vi "Ridders Zero Inner Part.vi"(0 "start/end/f(x)":T1 {"end" format="%.2f"; "start" format="%.2f"; "y value copy" format="%.2f"; "y value" format="%.2f"}, 1 "list of variables":i32[](array[numeric]), 2 "table":i32[][](array[numeric]), 3 "result":dbl[](array[numeric]) format="%.2f", 4 "accuracy":dbl format="%.2f", 5 "case":bool) -> (6 "y value":dbl format="%.2f", 7 "end":dbl format="%.2f", 8 "error":i32)   [LabVIEW 2010, in "NI_Gmath.lvlib"]
uses:
  NI_Gmath.lvlib
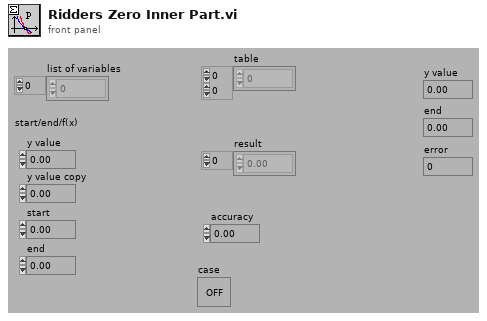
[diagram p1: front panel]
types:
  T1 = cluster{"y value":dbl, "y value copy":dbl, "start":dbl, "end":dbl}
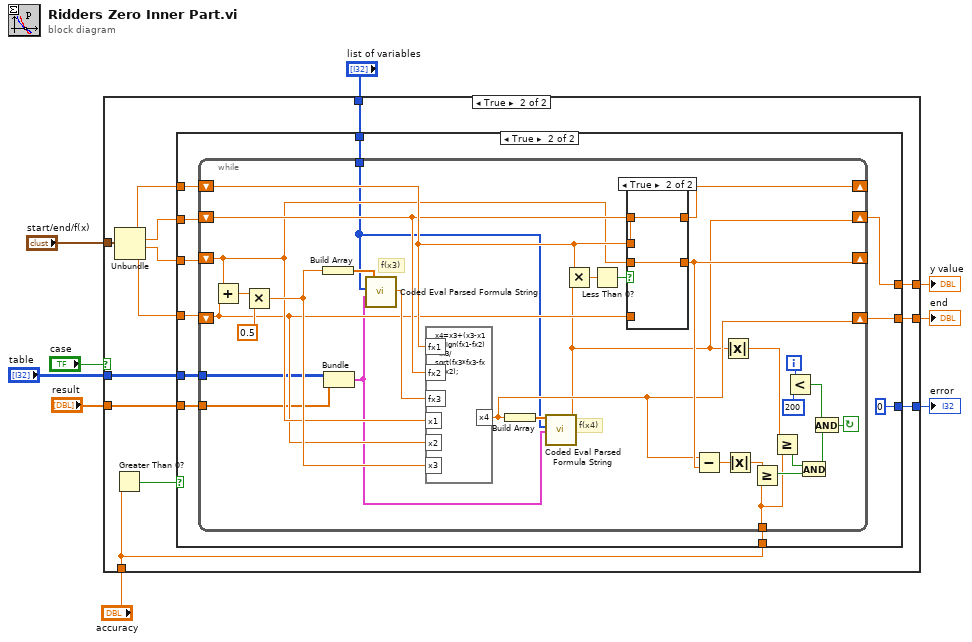
[diagram p0: block diagram]
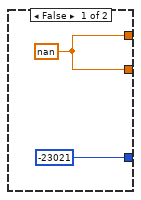
[diagram p2: hidden frame]
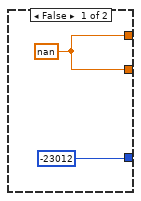
[diagram p3: hidden frame]
diagram:
  n1 = case shown="True" "case" {
    tunnel: [-23021 w23] -> w2
    tunnel: "accuracy" -> [_ w17]
    tunnel: [w10 w22] -> w4
    tunnel: [w10 w21] -> w5
    tunnel: "list of variables" -> [_ w20]
    tunnel: "table" -> [_ w19]
    tunnel: "result" -> [_ w18]
    tunnel: "start/end/f(x)" -> [_ w16]
    frame False {
      w10 = nan
    }
    frame True {
      n2 = Greater Than 0?(x=w17) -> (x > 0?=w24:bool)
      n3 = Unbundle(w16) -> ("y value"=w12:dbl, "y value copy"=w13:dbl, "start"=w14:dbl, "end"=w15:dbl)
      n4 = case shown="True" w24 {
        tunnel: w17 -> [_ w37]
        tunnel: w12 -> [_ w36]
        tunnel: w13 -> [_ w35]
        tunnel: w14 -> [_ w34]
        tunnel: w15 -> [_ w33]
        tunnel: [-23012 0] -> w23
        tunnel: [w25 w31] -> w22
        tunnel: [w25 w30] -> w21
        tunnel: w20 -> [_ w29]
        tunnel: w19 -> [_ w28]
        tunnel: w18 -> [_ w27]
        frame False {
          w25 = nan
        }
        frame True {
          n5 = while {
            tunnel: w27 -> [w39]
            tunnel: w28 -> [w41]
            tunnel: w29 -> [w40]
            tunnel: w37 -> [w51]
            shift-left: w35 -> [w62]
            shift-right: [w38] -> w30
            shift-left: w36 -> [w64]
            shift-right: [w63] -> _
            shift-left: w33 -> [w52]
            shift-right: [w50] -> w31
            shift-left: w34 -> [w53]
            shift-right: [w61] -> _
            i -> [w49]
            stop <- w46 continue-if-true
            # "f(x4)"
            # "f(x3)"
            n6 = Add(x=w53, y=w52) -> (x+y=w67:dbl)
            n7 = Multiply(x=w67, y=0.5) -> (x*y=w54:dbl)
            n8 = Build Array(w54) -> (w44:dbl[])
            n9 = Bundle("table"=w41, "result"=w39) -> (w43:cluster{"table":i32[][], "result":dbl[]})  [unwired: 1 in]
            n10 = call "Coded Eval Parsed Formula String.vi"("Parsed Formula"=w43, "Variables"=w40, "X Values"=w44) -> ("y value"=w55:dbl)  [unwired: 1 in, 1 out]
            n11 = formula code="x4=x3+(x3-x1)*sign(fx1-fx2)*fx3/sqrt(fx3*fx3-fx1*fx2);"("fx1"=w64, "fx2"=w62, "fx3"=w55, "x1"=w53, "x2"=w52, "x3"=w54) -> ("x4"=w50:dbl)
            n12 = Build Array(w50) -> (w42:dbl[])
            n13 = call "Coded Eval Parsed Formula String.vi"("Parsed Formula"=w43, "Variables"=w40, "X Values"=w42) -> ("y value"=w38:dbl)  [unwired: 1 in, 1 out]
            n14 = Multiply(x=w64, y=w38) -> (x*y=w66:dbl)
            n15 = Less Than 0?(x=w66) -> (x < 0?=w65:bool)
            n16 = case shown="True" w65 {
              tunnel: w53 -> [_ w72]
              tunnel: [w70 w72] -> w61
              tunnel: w52 -> [w70 _]
              tunnel: w64 -> [_ w71]
              tunnel: [w69 w71] -> w63
              tunnel: w62 -> [w69 _]
              frame False {
              }
              frame True {
              }
            }
            n17 = Subtract(x=w50, y=w61) -> (x-y=w59:dbl)
            n18 = Absolute Value(x=w38) -> (abs(x)=w58:dbl)
            n19 = Absolute Value(x=w59) -> (abs(x)=w60:dbl)
            n20 = Greater Or Equal?(x=w60, y=w51) -> (x >= y?=w56:bool)
            n21 = Greater Or Equal?(x=w58, y=w51) -> (x >= y?=w57:bool)
            n22 = Less?(x=w49, y=200) -> (x < y?=w47:bool)
            n23 = And(x=w57, y=w56) -> (x .and. y?=w45:bool)
            n24 = And(x=w47, y=w45) -> (x .and. y?=w46:bool)
          }
        }
      }
    }
  }
  "y value" <- w5
  "end" <- w4
  "error" <- w2
